vi "_Debug_LOGfilewrite344.vi"(7 "N":dbl, 8 "344cur":dbl, 9 "DAC1cur":dbl, 10 "DAC1volt2":dbl, 11 "refnum out":refnum<file>) -> ()   [LabVIEW 2017]
uses:
  <vilib>/Utility/error.llb/whitespace.ctl
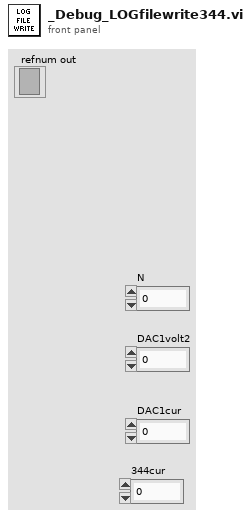
[diagram p1: front panel]
types:
  T1 = typedef "whitespace.ctl" = u16
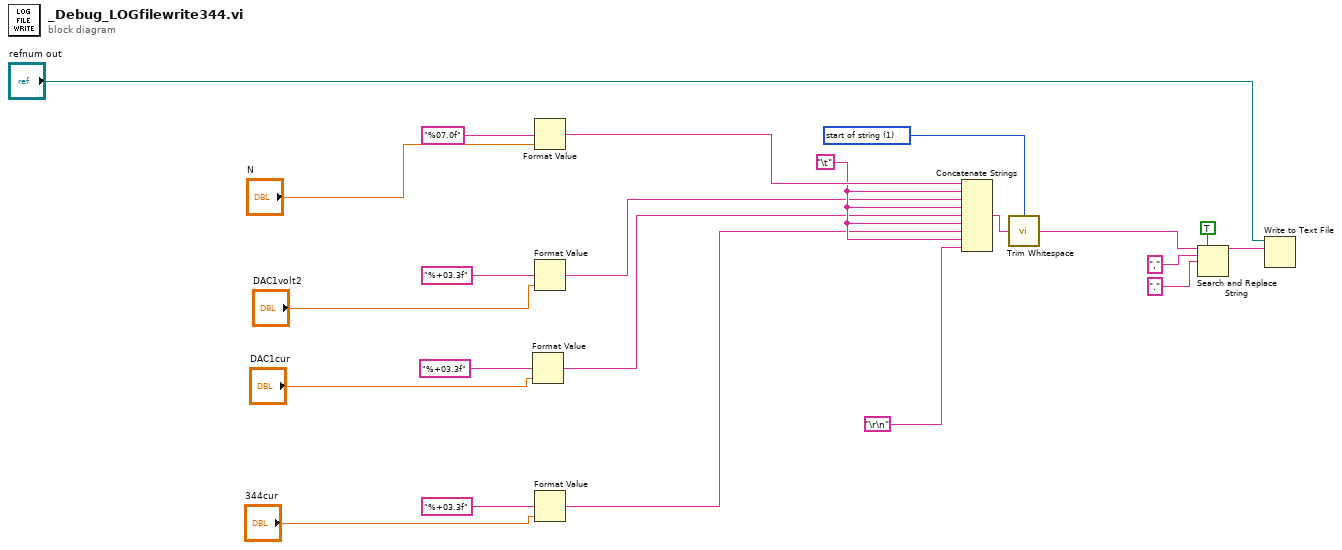
[diagram p0: block diagram]
diagram:
  w9 = "\t"
  w19 = T1 1 items=["both", "start of string", "end of string"] ("location (both)")
  n1 = Format Value(format string="%+03.3f", value (0)="DAC1cur") -> (output string=w5:string)  [unwired: 1 in]
  n2 = Format Value(format string="%07.0f", value (0)="N") -> (output string=w18:string)  [unwired: 1 in]
  n3 = Format Value(format string="%+03.3f", value (0)="DAC1volt2") -> (output string=w6:string)  [unwired: 1 in]
  n4 = Format Value(format string="%+03.3f", value (0)="344cur") -> (output string=w4:string)  [unwired: 1 in]
  n5 = Concatenate Strings(w18, w9, w6, w9, w5, w9, w4, w9, "\r\n") -> (w20:string)
  n6 = call <vilib>:"Trim Whitespace.vi"("string"=w20, "location (both)"=w19) -> ("trimmed string"=w14:string)
  n7 = Search and Replace String(replace all?=TRUE ("replace all? (F)"), input string=w14, search string=",", replace string="." ("replace string (\"\")")) -> (result string=w13:string)  [unwired: 4 in, 3 out]
  n8 = Write to Text File(file (use dialog)="refnum out", text=w13) -> ()  [unwired: 2 in, 3 out]
